vi "HRTF-Compute HRTF.vi"(0 "ear path":path, 1 "Window":T1, 7 "speaker path":path, 11 "Error In":errorcluster, 12 "Desired Fs":dbl) -> (15 "error out":errorcluster)   [LabVIEW 2015]
uses:
  Typedefs/HRTF-Window.ctl
  Typedefs/HRTF-Window Type.ctl
  Typedefs/HRTF-filt Cluster.ctl
  <vilib>/Analysis/2dsp.llb/Real FFT.vi
  <vilib>/Analysis/2dsp.llb/Inverse Real FFT.vi
  <vilib>/Analysis/2dsp.llb/Rational Resample (single channel, DBL).vi
  <userlib>/_matio/level5/Public/Write/Append Data Element.llb/Append Data Element (Anything).vi
  <vilib>/Analysis/NI_AALPro.lvlib
  <userlib>/_matio/level5.lvlib
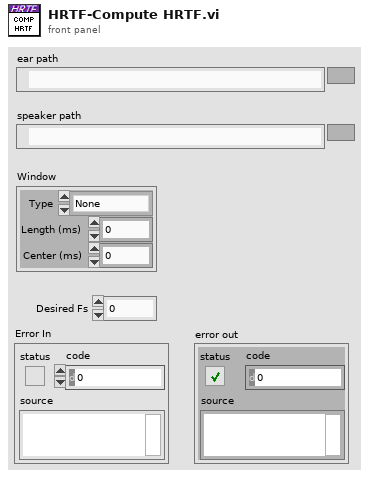
[diagram p1: front panel]
types:
  T1 = typedef "HRTF-Window.ctl" = cluster{"Type":T2, "Length (ms)":dbl, "Center (ms)":dbl}
  T2 = typedef "HRTF-Window Type.ctl" = enum16{"None", "Rectangle", "Hanning"}
  T3 = enum16{"big-endian, network order", "native, host order", "little-endian"}
  T4 = typedef "HRTF-filt Cluster.ctl" = cluster{"Type":string, "Fs":dbl, "a":dbl[], "b":dbl[], "window":i32, "Length_ms":dbl, "Center_ms":dbl}
  T5 = typedef "HRTF-Parameters.ctl" = cluster{"Fs (Hz)":dbl, "atten (dB)":dbl, "Waveform":T6, "Freq Res (Hz)":dbl, "Order":i32, "Averages":i32, "seed":i64, "Window":T1}
  T6 = typedef "HRTF-Waveform.ctl" = enum16{"Chirp", "MLS"}
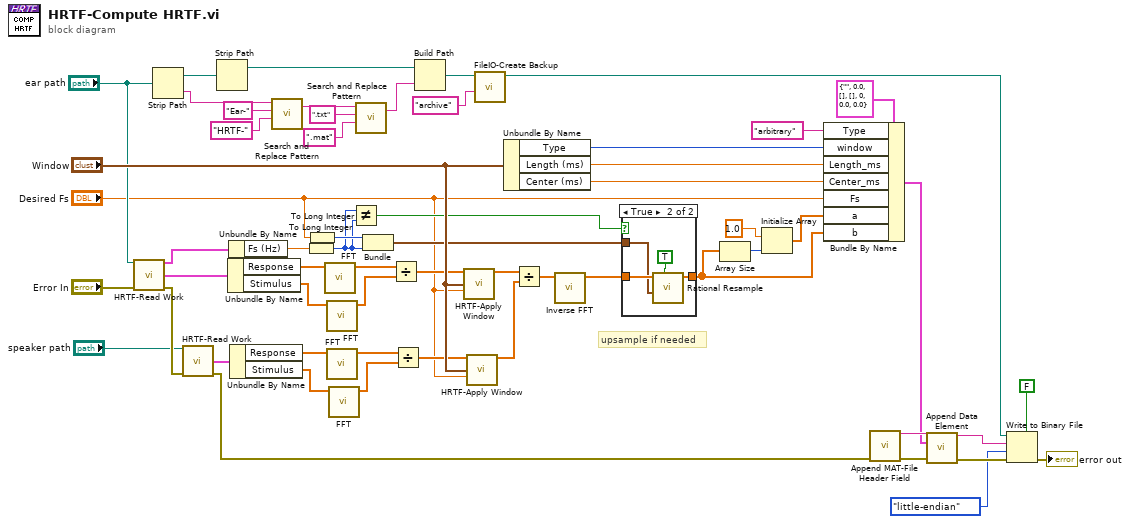
[diagram p0: block diagram]
diagram:
  # "upsample if needed"
  n1 = call "HRTF-Read Work.vi"("path"="ear path", "Error In"="Error In") -> ("Params"=w49:T5, "Result"=w58:cluster{"Stimulus":dbl[], "Response":dbl[]}, "error out"=w50:errorcluster)  [unwired: 11 in]
  n2 = Strip Path(path="ear path") -> (stripped path=w33:path, name=w32:string)
  n3 = call "HRTF-Read Work.vi"("path"="speaker path", "Error In"=w50) -> ("Result"=w53:cluster{"Stimulus":dbl[], "Response":dbl[]}, "error out"=w44:errorcluster)  [unwired: 11 in, 1 out]
  n4 = Strip Path(path=w33) -> (stripped path=w26:path)  [unwired: 1 out]
  n5 = Unbundle By Name(w58) -> ("Response"=w13:dbl[], "Stimulus"=w12:dbl[])
  n6 = Unbundle By Name(w49) -> ("Fs (Hz)"=w7:dbl)
  n7 = Unbundle By Name(w53) -> ("Response"=w11:dbl[], "Stimulus"=w10:dbl[])
  n8 = call <vilib>:"Search and Replace Pattern.vi"("string"=w32, "regular expression (\"\")"="Ear-" ("regular expression (\"\")"), "replace string (\"\")"="HRTF-" ("regular expression (\"\")")) -> ("result string"=w29:string)  [unwired: 2 in, 1 out]
  n9 = To Long Integer(number=w7) -> (32bit integer=w3:i32)
  n10 = To Long Integer(number="Desired Fs") -> (32bit integer=w14:i32)
  n11 = call-poly <vilib>:"FFT.vi"("X"=w13) -> ("FFT {X}"=w57:cdb[])  [unwired: 9 in, 1 out]
  n12 = call-poly <vilib>:"FFT.vi"("X"=w12) -> ("FFT {X}"=w56:cdb[])  [unwired: 9 in, 1 out]
  n13 = call-poly <vilib>:"FFT.vi"("X"=w11) -> ("FFT {X}"=w55:cdb[])  [unwired: 9 in, 1 out]
  n14 = call-poly <vilib>:"FFT.vi"("X"=w10) -> ("FFT {X}"=w54:cdb[])  [unwired: 9 in, 1 out]
  n15 = Not Equal?(x=w3, y=w3) -> (x != y?=w2:bool)
  n16 = call <vilib>:"Search and Replace Pattern.vi"("string"=w29, "regular expression (\"\")"=".txt" ("regular expression (\"\")"), "replace string (\"\")"=".mat" ("replace string (\"\")")) -> ("result string"=w25:string)  [unwired: 2 in, 1 out]
  n17 = Bundle(w14, w3) -> (w4:cluster{i32, i32})  [unwired: 1 in]
  n18 = Divide(x=w57, y=w56) -> (x/y=w9:cdb[])
  n19 = Divide(x=w55, y=w54) -> (x/y=w8:cdb[])
  n20 = Build Path(base path=w26, name or relative path=w25) -> (appended path=w24:path)
  n21 = call "HRTF-Apply Window.vi"("Array in"=w9, "Window"="Window", "Fs (Hz)"="Desired Fs") -> ("Array out"=w35:cdb[])  [unwired: 12 in]
  n22 = call "HRTF-Apply Window.vi"("Array in"=w8, "Window"="Window", "Fs (Hz)"="Desired Fs") -> ("Array out"=w34:cdb[])  [unwired: 12 in]
  n23 = call "FileIO-Create Backup.vi"("Subfolder"="archive", "Path"=w24) -> ("Path (thru)"=w22:path)  [unwired: 6 in, 3 out]
  n24 = Unbundle By Name("Window") -> ("Type"=w19:T2, "Length (ms)"=w18:dbl, "Center (ms)"=w17:dbl)
  n25 = Divide(x=w35, y=w34) -> (x/y=w52:cdb[])
  n26 = call-poly <vilib>:"Inverse FFT.vi"("FFT {X}"=w52) -> ("X"=w6:dbl[])  [unwired: 9 in, 1 out]
  n27 = case shown="True" w2 {
    tunnel: w6 -> [w59 w63]
    tunnel: [w59 w62] -> w5
    tunnel: w4 -> [_ w61]
    frame False {
    }
    frame True {
      n28 = call-poly <vilib>:"Rational Resample.vi"("reset"=TRUE, "resample factor"=w61, "X"=w63) -> ("Y"=w62:dbl[])  [unwired: 6 in, 2 out]
    }
  }
  n29 = Array Size(array=w5) -> (size(s)=w46:i32)
  n30 = Initialize Array(1.0 ("element"), w46) -> (w47:dbl[])
  n31 = Bundle By Name(cluster=T4 {"Type"="", "Fs"=0.0, "a"=[], "b"=[], "window"=0, "Length_ms"=0.0, "Center_ms"=0.0} ("filt"), "Type"="arbitrary", "window"=w19, "Length_ms"=w18, "Center_ms"=w17, "Fs"="Desired Fs", "a"=w47, "b"=w5) -> (w41:T4)
  n32 = call <userlib>:"Append MAT-File Header Field.vi"("error"=w44) -> ("result string"=w42:string, "error out"=w43:errorcluster)  [unwired: 13 in]
  n33 = call-poly <userlib>:"Append Data Element.vi"("initial string"=w42, "data"=w41, "error in (no error)"=w43) -> ("result string"=w39:string, "error out"=w40:errorcluster)  [unwired: 11 in]
  n34 = Write to Binary File(file (use dialog)=w22, data=w39, error in=w40, 5:FALSE ("prepend array or string size? (T)"), 9:T3."little-endian" ("byte order (0:big-endian, network order)")) -> (error out=→"error out":errorcluster)  [unwired: 1 in, 2 out]
